vi "SPI Write Read 1 Frame.vi"(5 "CS Configuration":T1={"CS Channel"=10, "CS Logic Level"=enum."Active Low"}, 7 "SPI Channel (0)":u8, 8 "Error In":errorcluster, 10 "Data":u8[](array[numeric]), 11 "LINX Resource":T3) -> (0 "Error Out":errorcluster, 2 "Read Data":u8[](array[numeric]), 3 "LINX Resource":T3)   [LabVIEW 2011, in "LVH-LINX.lvlib"]
doc: "Write/Read the specified SPI channel. SPI is full duplex, therefore the write and read operations take place simultaneously.\n\n<b>SPI Channel</b> specifies the device SPI channel to write/read to.\n\n<b>Data</b> is a U8 array of data bytes to shift out starting with Data[0] to Data[n-1].\n\n<b>CS Channel</b> is the Chip Select (DIO) channel to use during the SPI transaction.\n\n<b>CS Logic Level</b> specifies the logic level of the CS pin. Active low is most common and means that CS will idle high, then be driven low when a frame begins. All Data bytes are shifted out, then CS will be driven high to end the frame."
uses:
  LVH-LINX.lvlib
  Private/Type Defs/LINX Ref.ctl
  Private/Type Defs/Platform.ctl
  Private/Type Defs/Interface.ctl
  Private/Device/Type Defs/LINX Device Config.ctl
  Private/Device/Type Defs/TCP Config.ctl
  Private/Device/Type Defs/Channels.ctl
  SPI CS Config.ctl
  Private/Type Defs/Peripherals/SPI/SPI CS Logic Level.ctl
  Private/Device/Device.lvlib
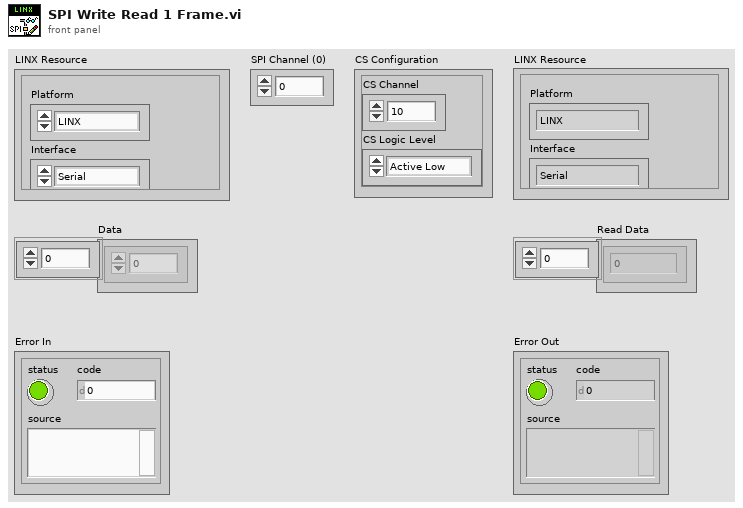
[diagram p1: front panel]
types:
  T1 = typedef "LVH-LINX.lvlib/SPI CS Config.ctl" = cluster{"CS Channel":u8, "CS Logic Level":T2}
  T2 = typedef "LVH-LINX.lvlib/SPI CS Logic Level.ctl" = enum8{"Active Low", "Active High"}
  T3 = typedef "LVH-LINX.lvlib/LINX Ref.ctl" = cluster{"Platform":T4, "Interface":T5, "LINX Device Config":T6}
  T4 = typedef "LVH-LINX.lvlib/Platform.ctl" = enum16{"LINX", "myRIO"}
  T5 = typedef "LVH-LINX.lvlib/Interface.ctl" = enum16{"Serial", "TCP"}
  T6 = typedef "LVH-LINX.lvlib/Device.lvlib/LINX Device Config.ctl" = cluster{"Interface":T5, "COM Port":refnum<visa-resource-name>, "TCP Configuration":T7, "Device Family":u8, "Device ID":u8, "Device Name":string, "TCP Ref":refnum<k5>, "Channels":T8}
  T7 = typedef "LVH-LINX.lvlib/Device.lvlib/TCP Config.ctl" = cluster{"IP Address":string, "Port":u16}
  T8 = typedef "LVH-LINX.lvlib/Channels.ctl" = cluster{"DI Channels":u8[], "DO Channels":u8[], "AI":u8[], "AO":u8[], "PWM":u8[], "QE":u8[], "UART":u8[], "I2C 2":u8[], "SPI":u8[], "CAN":u8[], "AI Ref (V)":dbl, "AO Resolution (Bits)":u8, "AO Ref (V)":dbl}
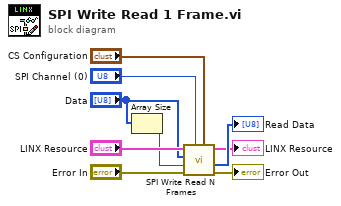
[diagram p0: block diagram]
diagram:
  n1 = Array Size(array="Data") -> (size(s)=w2:i32)
  n2 = call "SPI Write Read N Frames.vi"("CS Configuration"="CS Configuration", "SPI Channel (0)"="SPI Channel (0)", "Error In"="Error In", "SPI Frame Size (0)"=w2, "Data"="Data", "LINX Resource"="LINX Resource") -> ("Error Out"=→"Error Out":errorcluster, "Read Data"=→"Read Data":u8[], "LINX Resource"=→"LINX Resource":T3)  [unwired: 3 in]
